vi "Create G-CLI Sink.vi"(8 "error in (no error)":errorcluster, 11 "CLI Connection":refnum<class "CLI.lvclass">) -> (0 "error out":errorcluster)   [LabVIEW 2020, in "LV Logging.lvlib"]
uses:
  LV Logging.lvlib
  G-CLI Sink/G-CLI Sink.lvclass
  C:/Users/hughe_cx/Documents/LVLog/Source/File Sink/File Sink.lvclass
  C:/Users/hughe_cx/Documents/LVLog/Source/Sink/Sink.lvclass
  C:/Users/hughe_cx/Documents/LVLog/Source/G-CLI Sink/G-CLI Sink.lvclass
  <vilib>/Wiresmith Technology/G CLI/CLI Class/CLI.lvclass
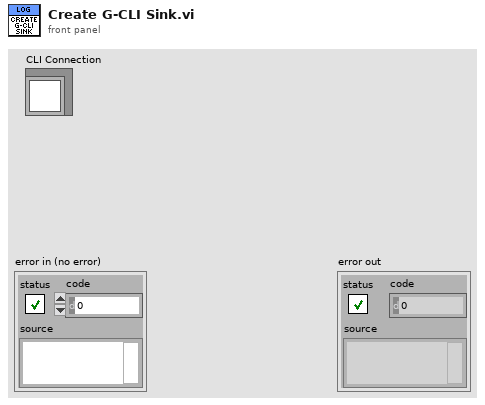
[diagram p1: front panel]
types:
  T1 = enum16{"Init", "Get Logger", "Register Sink", "Set Global Debug Level", "Get Sinks"}
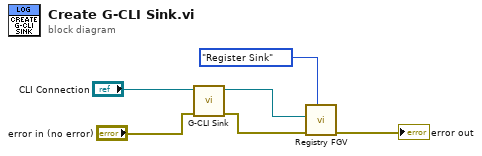
[diagram p0: block diagram]
diagram:
  n1 = call "G-CLI Sink.vi"("error in (no error)"="error in (no error)", "CLI Connection"="CLI Connection") -> ("error out"=w3:errorcluster, "G-CLI Sink out"=w2:refnum<class "G-CLI Sink.lvclass">)  [unwired: 8 in]
  n2 = call "Registry FGV.vi"("State (Get Logger)"=T1."Register Sink", "error in (no error)"=w3, "Sink"=w2) -> ("error out"=→"error out":errorcluster)  [unwired: 5 in, 3 out]
